vi "Sync outputs.vi"(4 "error in (no error)":errorcluster, 6 "Output image":u8[](array[numeric]), 7 "CANopen in":refnum<class "CANopen.lvclass">) -> (0 "error out":errorcluster, 2 "Changed?":bool, 3 "CANopen out":refnum<class "CANopen.lvclass">)   [LabVIEW 2017, in "canopen.lvlib" / "CANopen.lvclass"]
doc: "Synchronizes the provided output image with the internal one by sending a serie of RxPDO messages. The image is expected to contain the data mapped with \"Set output map\"."
uses:
  CANopen.lvclass
  CANopen.lvclass/CANopen.ctl
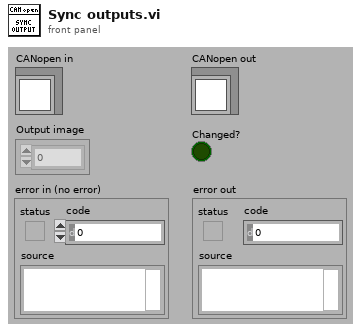
[diagram p1: front panel]
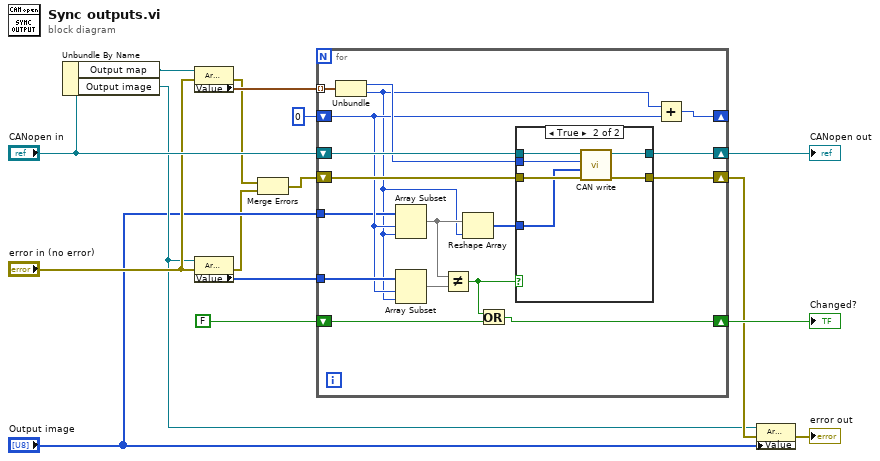
[diagram p0: block diagram]
diagram:
  n1 = Unbundle By Name("CANopen in") -> ("Output map"=w14:refnum<vi>, "Output image"=w5:refnum<vi>)
  n2 = property class="Arr (strict)"(reference=w14, error in="error in (no error)") -> (error out=w2:errorcluster, "Value"=w15:cluster{"CobID":u32, "nBytes":u8}[])  [unwired: 1 out]
  n3 = property class="Arr (strict)"(reference=w5, error in="error in (no error)") -> (error out=w3:errorcluster, "Value"=w8:u8[])  [unwired: 1 out]
  n4 = Merge Errors(w2, w3) -> (w1:errorcluster)
  n5 = for {
    tunnel: w15 -> [w33] mode=indexing
    shift-right: [w32] -> _
    shift-left: 0 -> [w25]
    shift-right: [w29] -> w7
    shift-left: w1 -> [w28]
    shift-right: [w22] -> w11
    shift-left: FALSE ("Changed?") -> [w23]
    tunnel: w8 -> [w26]
    tunnel: "Output image" -> [w20]
    shift-right: [w30] -> w13
    shift-left: "CANopen in" -> [w31]
    n6 = Unbundle(w33) -> ("CobID"=w27:u32, "nBytes"=w17:u8)
    n7 = Array Subset(array=w20, index=w25, length=w17) -> (w19:u8[])
    n8 = Array Subset(array=w26, index=w25, length=w17) -> (w24:u8[])
    n9 = Not Equal?(x=w19, y=w24) -> (x != y?=w21:bool)
    n10 = Reshape Array(w19, w17) -> (w18:u8[])
    n11 = Or(x=w21, y=w23) -> (x .or. y?=w22:bool)
    n12 = case shown="True" w21 {
      tunnel: w31 -> [w34 w41]
      tunnel: [w34 w40] -> w30
      tunnel: [w35 w39] -> w29
      tunnel: w28 -> [w35 w38]
      tunnel: w27 -> [_ w37]
      tunnel: w18 -> [_ w36]
      frame False {
      }
      frame True {
        n13 = call "CAN write.vi"("error in (no error)"=w38, "Data"=w36, "COB id"=w37, "CANopen in"=w41) -> ("error out"=w39:errorcluster, "CANopen out"=w40:refnum<class "CANopen.lvclass">)  [unwired: 2 out]
      }
    }
    n14 = Add(x=w17, y=w25) -> (x+y=w32:i32)
  }
  "Changed?" <- w11
  "CANopen out" <- w13
  n15 = property class="Arr (strict)"(reference=w5, error in=w7, "Value"="Output image") -> (error out=→"error out":errorcluster)  [unwired: 1 out]
